vi "POST_control.vi"(7 "LabVIEW Web Service Request":refnum<class "Web Request.lvclass">) -> ()   [LabVIEW 2019]
uses:
  <vilib>/wsapi/Web Request.lvclass
panel:
  out "postdata":string
  # "Use the Web Service Request input terminal to call the VIs on the Web Services palette. Do not remove it from the connector pane unless you don't need access to the palette."
  # "Each additional control wired to the connector pane will be available as an input in the URL. To include an indicator in terminal-mode output (the default setting), it must also be wired to the connector pane."
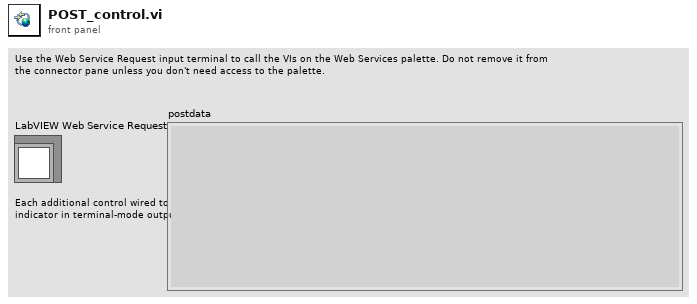
[diagram p1: front panel]
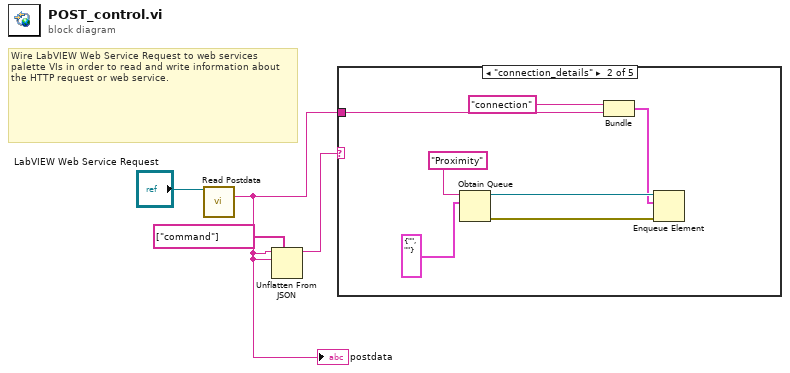
[diagram p0: block diagram]
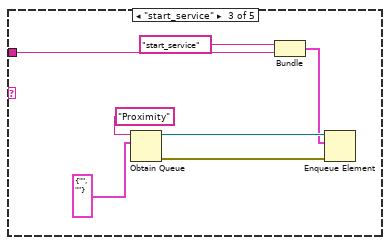
[diagram p3: hidden frame]
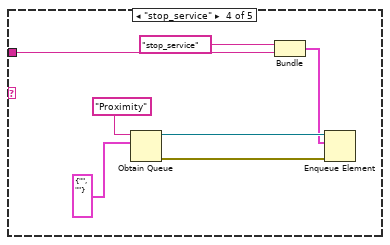
[diagram p4: hidden frame]
diagram:
  # "Wire LabVIEW Web Service Request to web services palette VIs in order to read and write information about the HTTP request or web service."
  n1 = call <vilib>:"Read Postdata.vi"("LabVIEW Web Service Request"="LabVIEW Web Service Request") -> ("postdata"=w2:string)  [unwired: 12 in, 2 out]
  "postdata" <- w2
  n2 = Unflatten From JSON(path=string[] ["command"], JSON string=w2, type and defaults=w2) -> (value=w1:string)  [unwired: 4 in, 1 out]
  n3 = case shown="\"connection_details\"" w1 {
    tunnel: w2 -> [_ w5 w12 w19 _]
    frame Default {
    }
    frame "connection_details" {
      n4 = Obtain Queue(name (unnamed)="Proximity", element data type=cluster{string, "postdata":string} {"", "postdata"=""} ("output cluster")) -> (queue out=w10:refnum<queue>, error out=w9:errorcluster)  [unwired: 3 in, 1 out]
      n5 = Bundle("connection", "postdata"=w5) -> (w7:cluster{string, "postdata":string})  [unwired: 1 in]
      n6 = Enqueue Element(queue=w10, element=w7, error in (no error)=w9) -> ()  [unwired: 1 in, 3 out]
    }
    frame "start_service" {
      n7 = Obtain Queue(name (unnamed)="Proximity", element data type=cluster{string, "postdata":string} {"", "postdata"=""} ("output cluster")) -> (queue out=w17:refnum<queue>, error out=w16:errorcluster)  [unwired: 3 in, 1 out]
      n8 = Bundle("start_service", "postdata"=w12) -> (w14:cluster{string, "postdata":string})  [unwired: 1 in]
      n9 = Enqueue Element(queue=w17, element=w14, error in (no error)=w16) -> ()  [unwired: 1 in, 3 out]
    }
    frame "stop_service" {
      n10 = Obtain Queue(name (unnamed)="Proximity", element data type=cluster{string, "postdata":string} {"", "postdata"=""} ("output cluster")) -> (queue out=w24:refnum<queue>, error out=w23:errorcluster)  [unwired: 3 in, 1 out]
      n11 = Bundle("stop_service", "postdata"=w19) -> (w21:cluster{string, "postdata":string})  [unwired: 1 in]
      n12 = Enqueue Element(queue=w24, element=w21, error in (no error)=w23) -> ()  [unwired: 1 in, 3 out]
    }
    frame "get_status" {
    }
  }
